vi "RunStep.vi"(4 "syringe_volume_uL":dbl=1000.0, 5 "MessageQueues":T1, 6 "Experiment":string[][](array[string]), 7 "Current Step 2":refnum<vi>, 8 "Pump Class":refnum<k24>, 9 "Bias":refnum<vi>, 10 "TimeTrace":refnum<vi>, 11 "Analyte":refnum<vi>) -> ()   [LabVIEW 2024]
uses:
  MessageQueues.ctl
  <vilib>/httpClient/ClientHandle.ctl
  E:/CodeProjects/DEMPbot/ChannelAutomatorR2/PumpAdapter.exe
  PumpAdapter.exe
  <vilib>/httpClient/LabVIEWHTTPClient.lvlib
panel:
  out "DispenseToCellLimited2":string
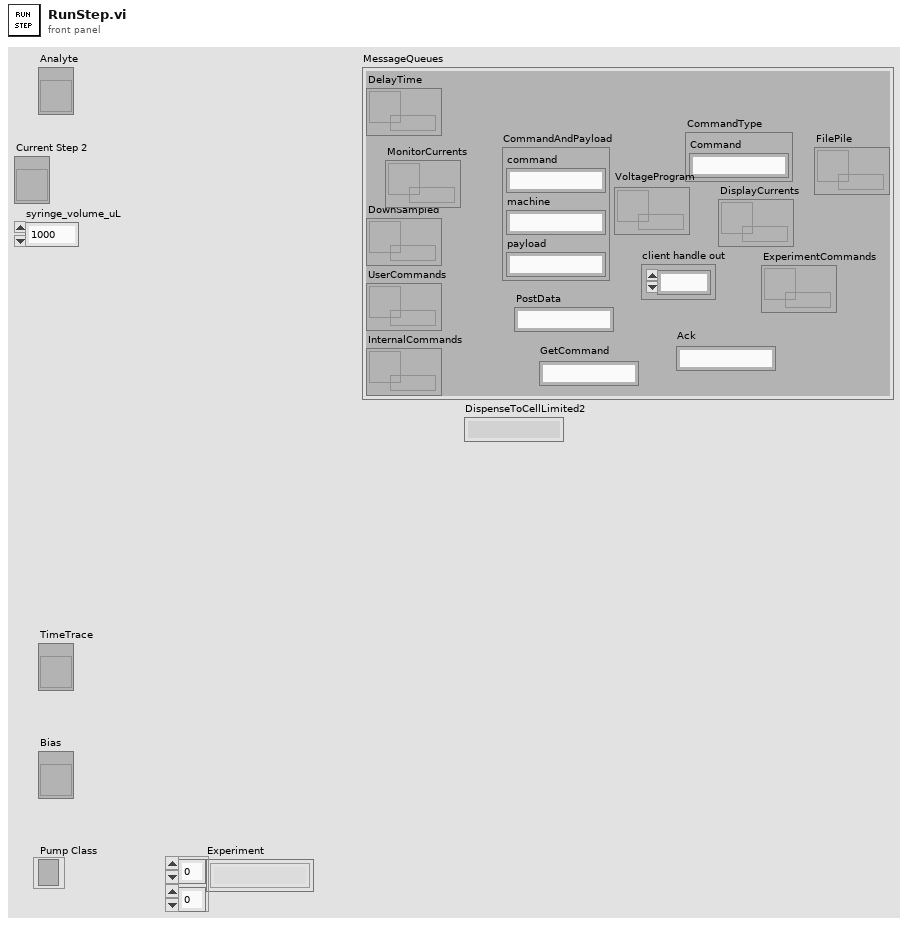
[diagram p1: front panel]
types:
  T1 = typedef "MessageQueues.ctl" = cluster{"DelayTime":refnum<queue>, "DownSampled":refnum<queue>, "UserCommands":refnum<queue>, "InternalCommands":refnum<queue>, "CommandType":cluster{"Command":string}, "CommandAndPayload":cluster{"command":string, "machine":string, "payload":string}, "client handle out":T2, "PostData":string, "GetCommand":string, "Ack":string, "VoltageProgram":refnum<queue>, "ExperimentCommands":refnum<queue>, "DisplayCurrents":refnum<queue>, "MonitorCurrents":refnum<queue>, "FilePile":refnum<queue>}
  T2 = typedef "LabVIEWHTTPClient.lvlib/ClientHandle.ctl" = refnum<k1>
  T3 = cluster{"Step":string, "Push":string, "Analyte1":string, "Volume1":dbl, "Analyte2":string, "Measurement":string, "Volume2":dbl, "Speed1":dbl, "Speed2":dbl, "MinTime":dbl, "Bias":dbl, "Slew":dbl, "Parameter1":string, "Parameter2":string}
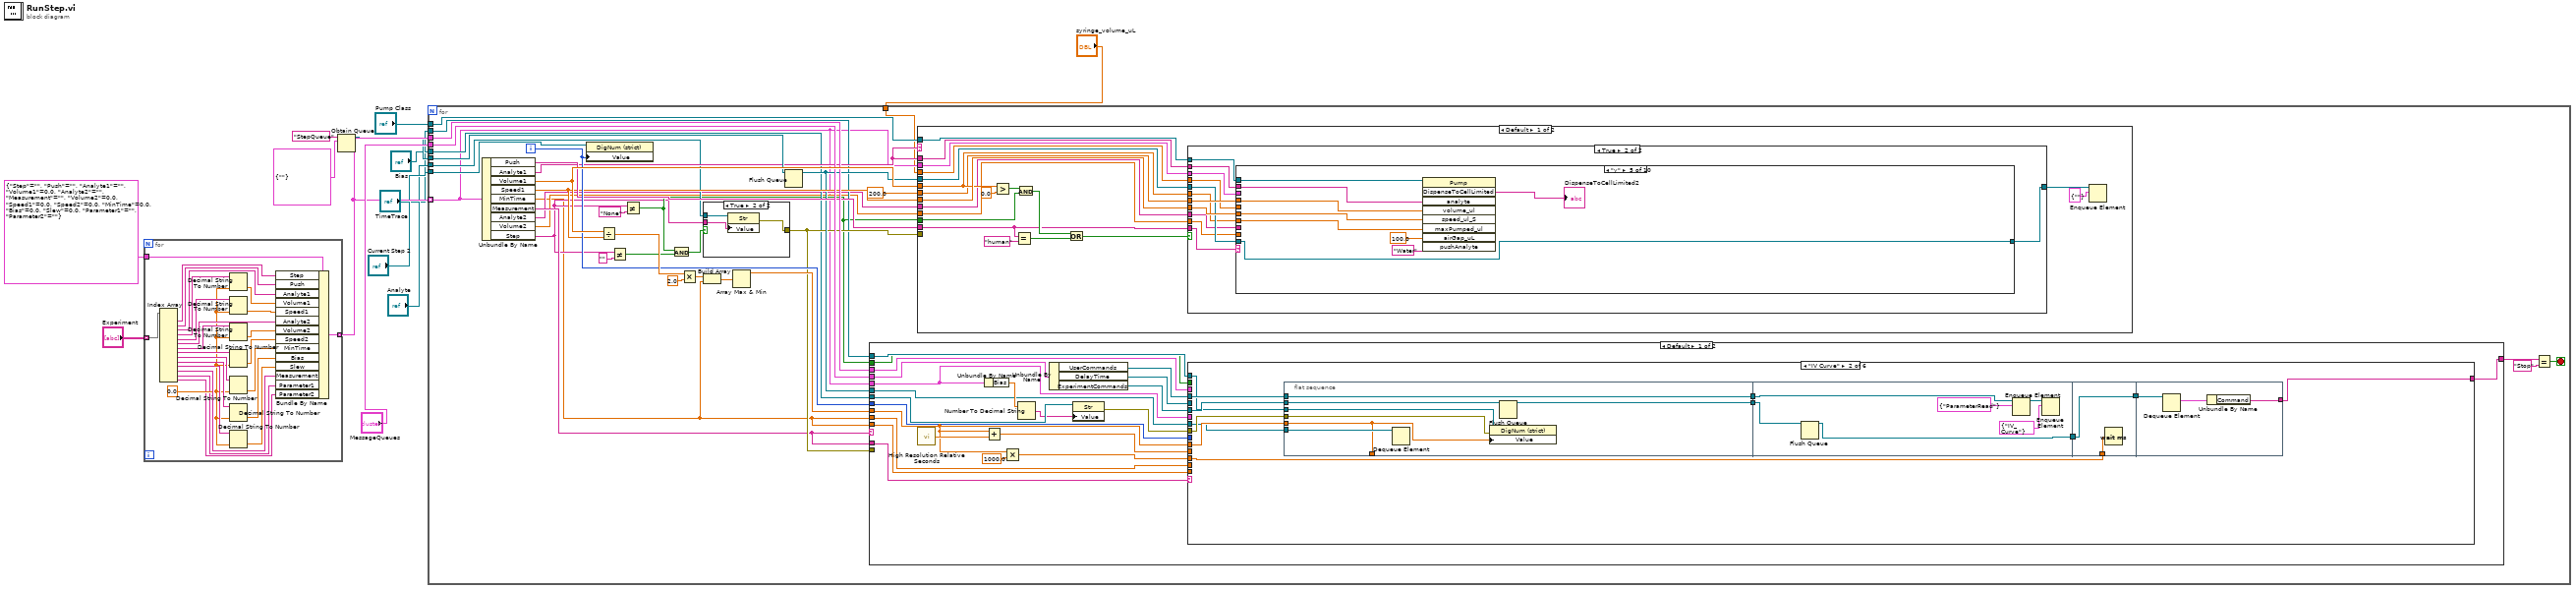
[diagram p0: block diagram]
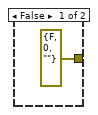
[diagram p2: hidden frame]
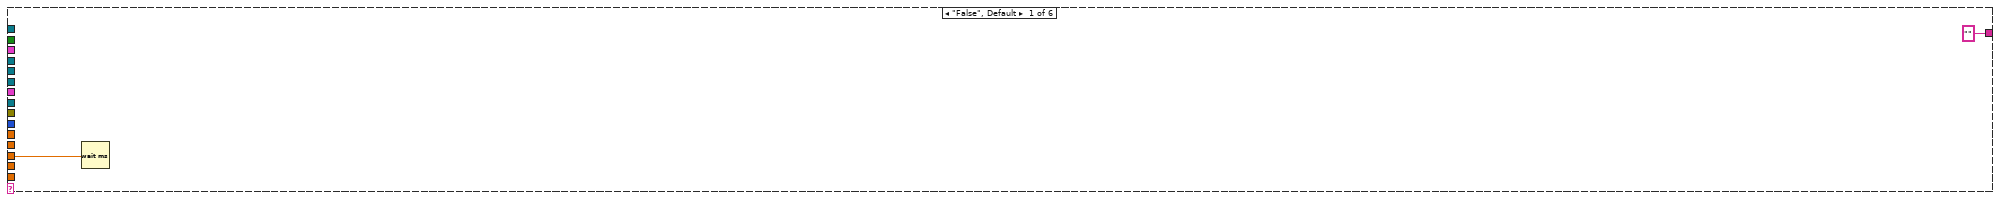
[diagram p3: hidden frame]
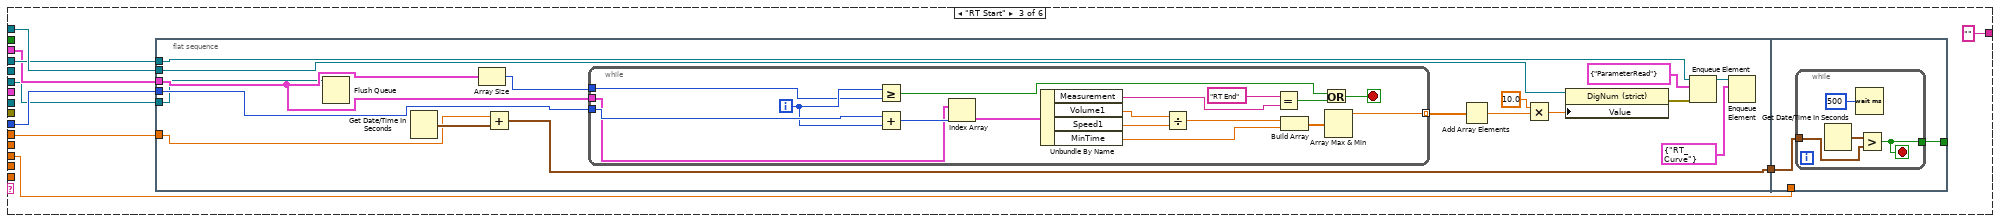
[diagram p4: hidden frame]
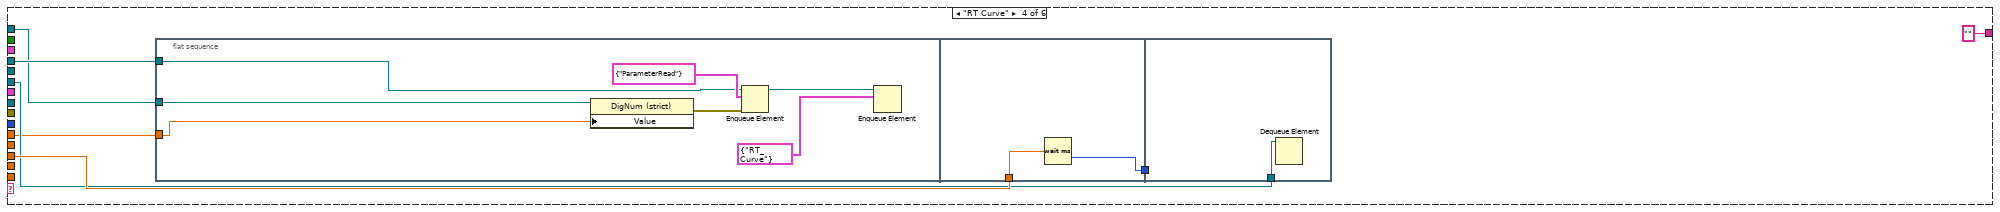
[diagram p5: hidden frame]
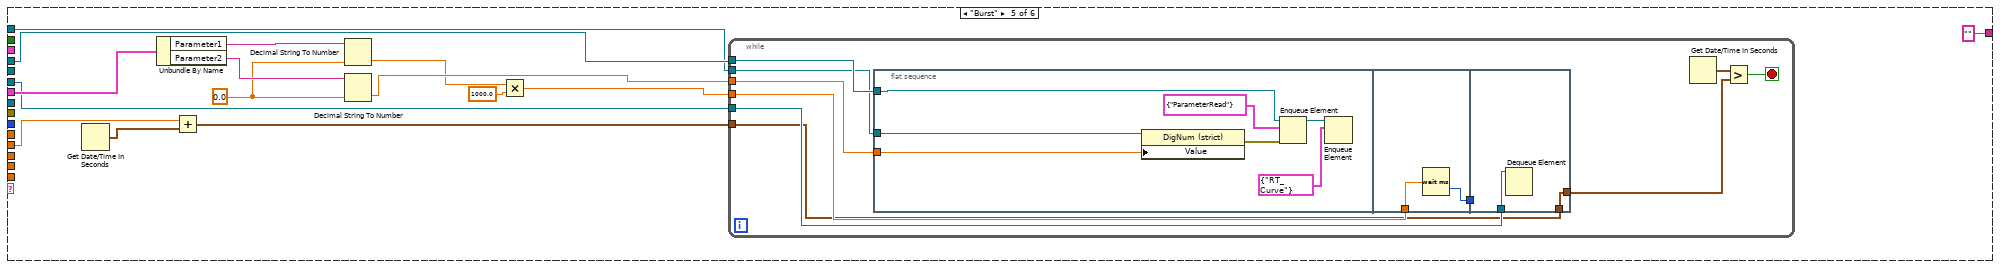
[diagram p6: hidden frame]
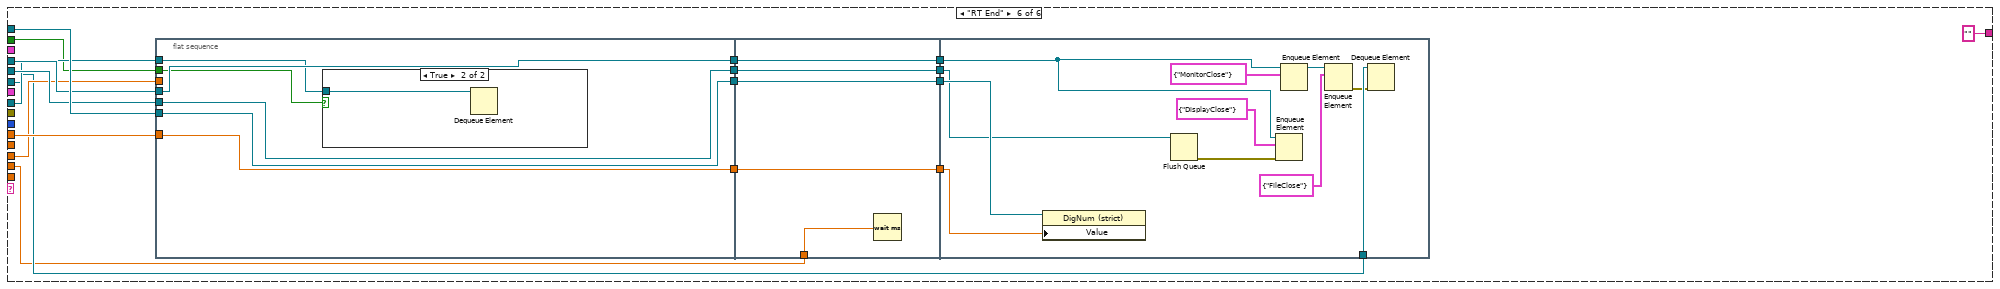
[diagram p7: hidden frame]
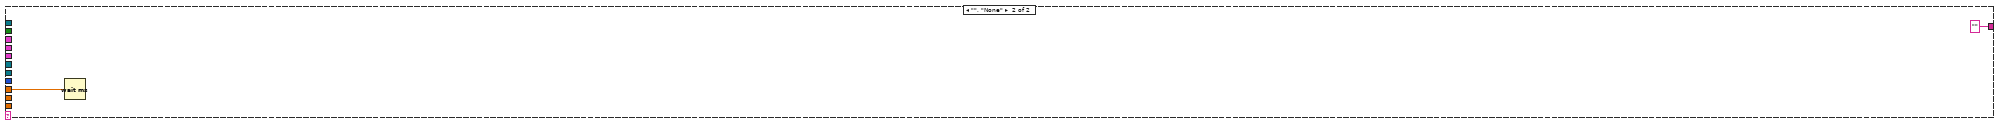
[diagram p9: hidden frame]
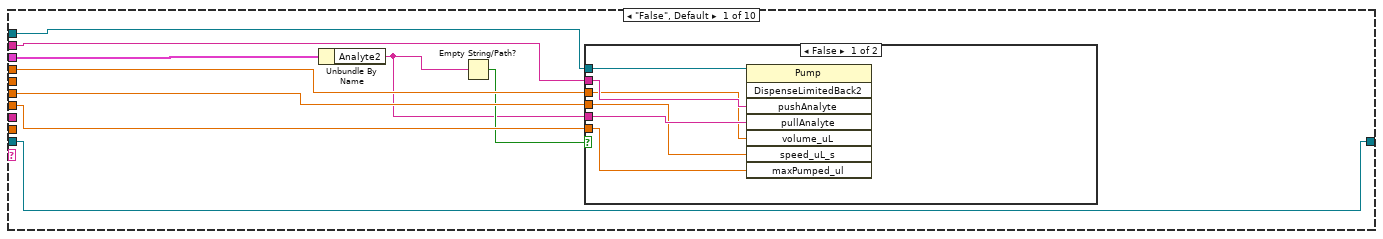
[diagram p11: hidden frame]
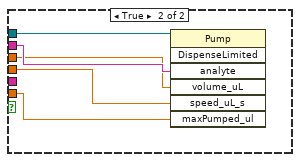
[diagram p12: hidden frame]
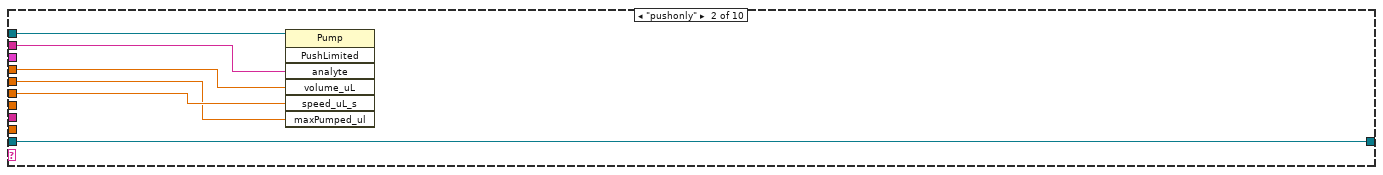
[diagram p13: hidden frame]
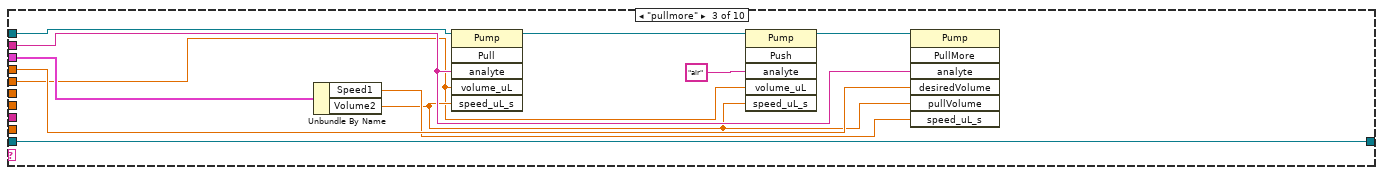
[diagram p14: hidden frame]
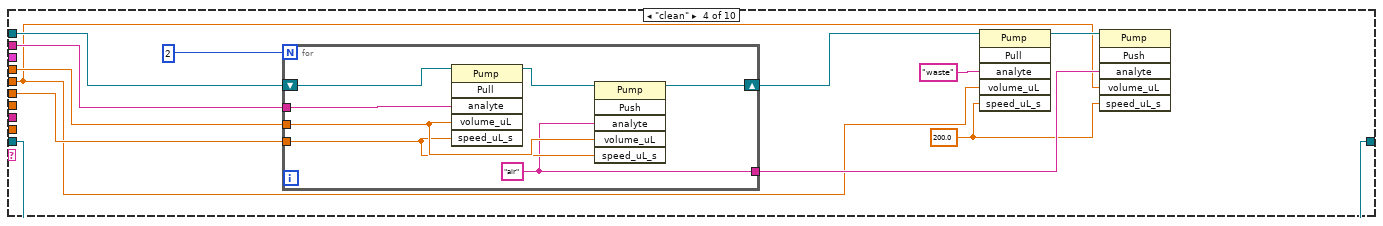
[diagram p15: hidden frame]
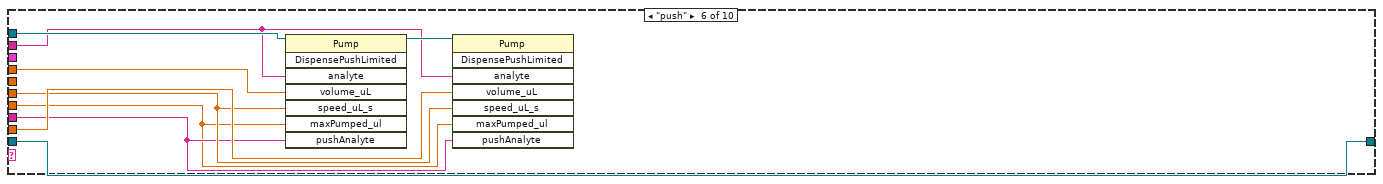
[diagram p16: hidden frame]
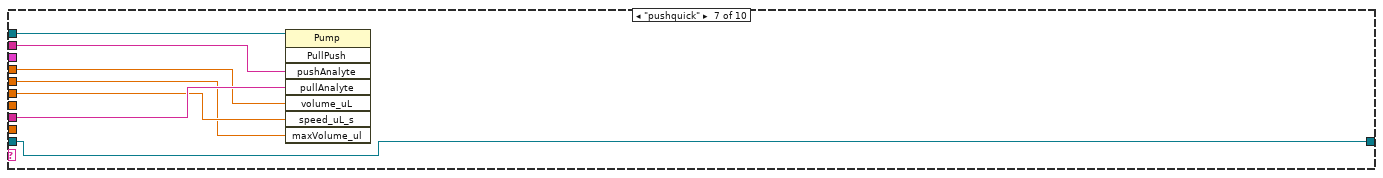
[diagram p17: hidden frame]
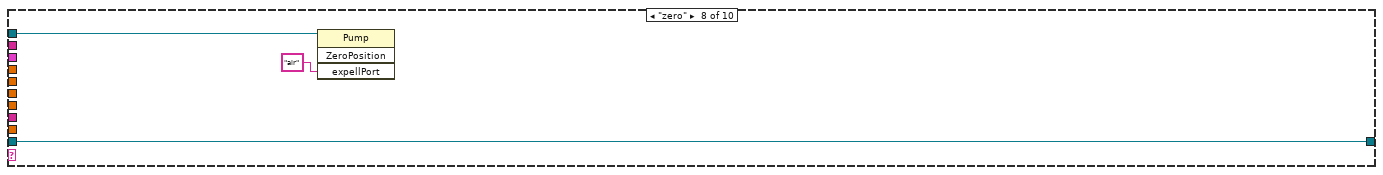
[diagram p18: hidden frame]
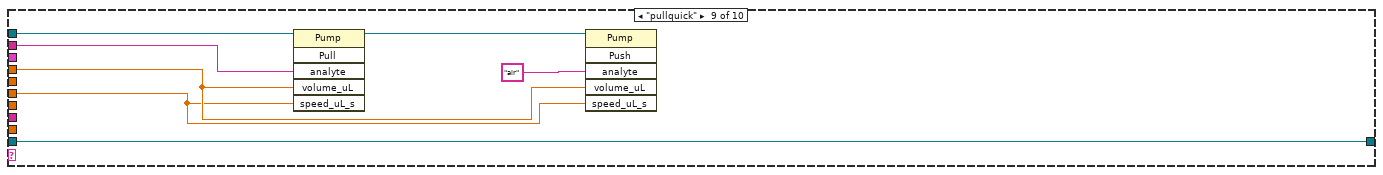
[diagram p19: hidden frame]
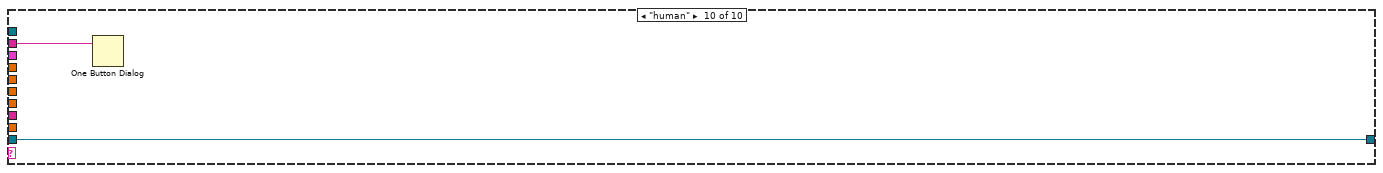
[diagram p20: hidden frame]
diagram:
  n1 = for {
    tunnel: T3 {"Step"="", "Push"="", "Analyte1"="", "Volume1"=0.0, "Analyte2"="", "Measurement"="", "Volume2"=0.0, "Speed1"=0.0, "Speed2"=0.0, "MinTime"=0.0, "Bias"=0.0, "Slew"=0.0, "Parameter1"="", "Parameter2"=""} -> [w19]
    tunnel: "Experiment" -> [w17] mode=indexing
    tunnel: [w16] -> w10 mode=indexing
    w20 = 0.0
    n2 = Index Array(array=w17) -> (element #1=w38:string, element #2=w37:string, element #3=w30:string, element #4=w36:string, element #5=w35:string, element #6=w34:string, element #7=w33:string, element #8=w32:string, element #9=w31:string, element #10=w28:string, element #11=w24:string, element #12=w23:string, element #13=w15:string, element #14=w14:string)  [unwired: 14 in]
    n3 = Decimal String To Number(string=w36, default (0L)=w20) -> (number=w25:dbl)  [unwired: 1 in, 1 out]
    n4 = Decimal String To Number(string=w35, default (0L)=w20) -> (number=w26:dbl)  [unwired: 1 in, 1 out]
    n5 = Decimal String To Number(string=w33, default (0L)=w20) -> (number=w27:dbl)  [unwired: 1 in, 1 out]
    n6 = Decimal String To Number(string=w32, default (0L)=w20) -> (number=w29:dbl)  [unwired: 1 in, 1 out]
    n7 = Decimal String To Number(string=w31, default (0L)=w20) -> (number=w18:dbl)  [unwired: 1 in, 1 out]
    n8 = Decimal String To Number(string=w28, default (0L)=w20) -> (number=w22:dbl)  [unwired: 1 in, 1 out]
    n9 = Decimal String To Number(string=w24, default (0L)=w20) -> (number=w21:dbl)  [unwired: 1 in, 1 out]
    n10 = Bundle By Name(cluster=w19, "Step"=w38, "Push"=w37, "Analyte1"=w30, "Volume1"=w25, "Speed1"=w26, "Analyte2"=w34, "Volume2"=w27, "Speed2"=w29, "MinTime"=w18, "Bias"=w22, "Slew"=w21, "Measurement"=w23, "Parameter1"=w15, "Parameter2"=w14) -> (w16:T3)
  }
  n11 = Obtain Queue(name (unnamed)="StepQueue", element data type=cluster{string} {""}) -> (queue out=w7:refnum<queue>)  [unwired: 3 in, 2 out]
  n12 = for {
    tunnel: "MessageQueues" -> [w70]
    tunnel: w10 -> [w66]
    tunnel: w10 -> [w43] mode=indexing
    tunnel: w7 -> [w62]
    tunnel: "Current Step 2" -> [w57]
    tunnel: "Analyte" -> [w56]
    tunnel: "Pump Class" -> [w55]
    tunnel: "Bias" -> [w54]
    tunnel: "TimeTrace" -> [w53]
    tunnel: "syringe_volume_uL" -> [w39]
    i -> [w65]
    stop <- w68 stop-if-true
    n13 = Unbundle By Name(w43) -> ("Push"=w64:string, "Analyte1"=w60:string, "Volume1"=w72:dbl, "Speed1"=w63:dbl, "MinTime"=w42:dbl, "Measurement"=w51:string, "Analyte2"=w50:string, "Volume2"=w49:dbl, "Step"=w44:string)
    n14 = property class="DigNum (strict)"(reference=w57, "Value"=w65) -> ()  [unwired: 1 in, 2 out]
    n15 = Divide(x=w72, y=w63) -> (x/y=w71:dbl)
    n16 = Not Equal?(x=w44, y="") -> (x != y?=w46:bool)
    n17 = Not Equal?(x=w44, y="None") -> (x != y?=w52:bool)
    n18 = And(x=w52, y=w46) -> (x .and. y?=w47:bool)
    n19 = Multiply(x=w71, y=2.0) -> (x*y=w41:dbl)
    n20 = case shown="True" w47 {
      tunnel: w56 -> [_ w78]
      tunnel: w44 -> [_ w77]
      tunnel: [errorcluster {"status"=FALSE, "code"=0, "source"=""} ("error out") w76] -> w58
      frame False {
      }
      frame True {
        n21 = property class="Str"(reference=w78, "Value"=w77) -> (error out=w76:errorcluster)  [unwired: 1 in, 1 out]
      }
    }
    n22 = Build Array(w41, w42) -> (w73:dbl[])
    n23 = Array Max & Min(array=w73) -> (max value=w74:dbl)  [unwired: 3 out]
    n24 = Flush Queue(queue=w62) -> (queue out=w61:refnum<queue>)  [unwired: 1 in, 2 out]
    n25 = case shown="Default" w51 {
      tunnel: w70 -> [w101 _]
      tunnel: w51 -> [w100 _]
      tunnel: w74 -> [w85 w278]
      tunnel: w43 -> [w98 _]
      tunnel: w53 -> [w94 _]
      tunnel: w54 -> [w96 _]
      tunnel: [w89 "" ("Command")] -> w67
      tunnel: w66 -> [w87 _]
      tunnel: w65 -> [w86 _]
      tunnel: w61 -> [w82 _]
      tunnel: w42 -> [w81 _]
      tunnel: w58 -> [_ _]
      tunnel: w52 -> [w80 _]
      tunnel: w42 -> [w79 _]
      frame Default {
        n26 = call <vilib>:"High Resolution Relative Seconds.vi"() -> ("relative seconds"=w91:dbl)
        n27 = Unbundle By Name(w98) -> ("Bias"=w97:dbl)
        n28 = Add(x=w85, y=w91) -> (x+y=w90:dbl)
        n29 = Multiply(x=w85, y=1000.0) -> (x*y=w83:dbl)
        n30 = Number To Decimal String(number=w97) -> (decimal integer string=w95:string)  [unwired: 1 in]
        n31 = Unbundle By Name(w101) -> ("UserCommands"=w99:refnum<queue>, "DelayTime"=w92:refnum<queue>, "ExperimentCommands"=w88:refnum<queue>)
        n32 = property class="Str"(reference=w96, "Value"=w95) -> (error out=w93:errorcluster)  [unwired: 1 in, 1 out]
        n33 = case shown="\"IV Curve\"" w100 {
          tunnel: w99 -> [_ w115 w141 w188 w209 w250]
          tunnel: w98 -> [_ _ _ _ w214 _]
          tunnel: w94 -> [_ w110 w142 w184 w203 w253]
          tunnel: w93 -> [_ w109 _ _ _ _]
          tunnel: w92 -> [_ _ _ _ _ w251]
          tunnel: w90 -> [_ _ _ _ w202 _]
          tunnel: ["" ("Command") w114 "" ("Command") "" ("Command") "" ("Command") "" ("Command")] -> w89
          tunnel: w88 -> [_ w113 w134 w185 w204 w238]
          tunnel: w85 -> [_ w108 w135 w183 _ w249]
          tunnel: w87 -> [_ _ w139 _ _ _]
          tunnel: w86 -> [_ _ w138 _ _ _]
          tunnel: w83 -> [w102 w104 w137 w187 _ w248]
          tunnel: w82 -> [_ w107 _ _ _ w247]
          tunnel: w81 -> [_ _ _ _ _ _]
          tunnel: w80 -> [_ _ _ _ _ w237]
          tunnel: w79 -> [_ _ _ _ _ w236]
          frame "False", Default {
            n34 = Wait (ms)(milliseconds to wait=w102) -> ()  [unwired: 1 out]
          }
          frame "IV Curve" {
            n35 = flat-sequence {
              tunnel: w113 -> [w121]
              tunnel: w115 -> [w122]
              tunnel: [w122] -> w112
              tunnel: [w117] -> w111
              tunnel: w110 -> [w120]
              tunnel: w109 -> [w119]
              tunnel: w108 -> [w116]
              tunnel: w107 -> [w118]
              tunnel: [w116] -> _
              tunnel: w112 -> [w128]
              tunnel: w111 -> [w124]
              tunnel: [w123] -> w106
              tunnel: w106 -> [w130]
              tunnel: [w130] -> w105
              tunnel: w104 -> [w129]
              tunnel: [w131] -> w114
              tunnel: w105 -> [w132]
              frame #0 {
                n36 = Dequeue Element(queue=w118) -> ()  [unwired: 2 in, 4 out]
                n37 = property class="DigNum (strict)"(reference=w120, error in=w119, "Value"=w116) -> ()  [unwired: 2 out]
                n38 = Flush Queue(queue=w121) -> (queue out=w117:refnum<queue>)  [unwired: 1 in, 2 out]
              }
              frame #1 {
                n39 = Flush Queue(queue=w124) -> (queue out=w123:refnum<queue>)  [unwired: 1 in, 2 out]
                n40 = Enqueue Element(queue=w128, element=cluster{"Command":string} {"Command"="ParameterRead"}) -> (queue out=w127:refnum<queue>)  [unwired: 2 in, 2 out]
                n41 = Enqueue Element(queue=w127, element=cluster{"Command":string} {"Command"="IV_Curve"}) -> ()  [unwired: 2 in, 3 out]
              }
              frame #2 {
                n42 = Wait (ms)(milliseconds to wait=w129) -> ()  [unwired: 1 out]
              }
              frame #3 {
                n43 = Dequeue Element(queue=w132) -> (element=w133:cluster{"Command":string})  [unwired: 2 in, 3 out]
                n44 = Unbundle By Name(w133) -> ("Command"=w131:string)
              }
            }
          }
          frame "RT Start" {
            n45 = flat-sequence {
              tunnel: w142 -> [w156]
              tunnel: w141 -> [w155]
              tunnel: w139 -> [w153]
              tunnel: w138 -> [w154]
              tunnel: [w145] -> w136
              tunnel: w135 -> [w144]
              tunnel: w134 -> [w143]
              tunnel: w137 -> [_]
              tunnel: w136 -> [w178]
              tunnel: [w177] -> _
              frame #0 {
                n46 = Flush Queue(queue=w143) -> ()  [unwired: 1 in, 3 out]
                n47 = Get Date/Time In Seconds() -> (seconds since 1Jan1904=w146:timestamp)
                n48 = Array Size(array=w153) -> (size(s)=w152:i32)
                n49 = Add(x=w144, y=w146) -> (x+y=w145:timestamp)
                n50 = while {
                  tunnel: w154 -> [w176]
                  tunnel: w153 -> [w174]
                  tunnel: w152 -> [w171]
                  tunnel: [w160] -> w151 mode=indexing
                  i -> [w172]
                  stop <- w169 stop-if-true
                  n51 = Greater Or Equal?(x=w172, y=w171) -> (x >= y?=w170:bool)
                  n52 = Add(x=w176, y=w172) -> (x+y=w175:i32)
                  n53 = Index Array(array=w174, index=w175) -> (element=w173:T3)
                  n54 = Unbundle By Name(w173) -> ("Measurement"=w168:string, "Volume1"=w165:dbl, "Speed1"=w164:dbl, "MinTime"=w162:dbl)
                  n55 = Divide(x=w165, y=w164) -> (x/y=w163:dbl)
                  n56 = Equal?(x="RT End", y=w168) -> (x = y?=w166:bool)
                  n57 = Build Array(w163, w162) -> (w161:dbl[])
                  n58 = Or(x=w170, y=w166) -> (x .or. y?=w169:bool)
                  n59 = Array Max & Min(array=w161) -> (max value=w160:dbl)  [unwired: 3 out]
                }
                n60 = Add Array Elements(numeric array=w151) -> (sum=w150:dbl)
                n61 = Multiply(x=10.0, y=w150) -> (x*y=w148:dbl)
                n62 = property class="DigNum (strict)"(reference=w156, "Value"=w148) -> (error out=w149:errorcluster)  [unwired: 1 in, 1 out]
                n63 = Enqueue Element(queue=w155, element=cluster{"Command":string} {"Command"="ParameterRead"}, error in (no error)=w149) -> (queue out=w159:refnum<queue>)  [unwired: 1 in, 2 out]
                n64 = Enqueue Element(queue=w159, element=cluster{"Command":string} {"Command"="RT_Curve"}) -> ()  [unwired: 2 in, 3 out]
              }
              frame #1 {
                n65 = while {
                  tunnel: w178 -> [w180]
                  tunnel: [w179] -> w177
                  stop <- w179 stop-if-true
                  n66 = Get Date/Time In Seconds() -> (seconds since 1Jan1904=w181:timestamp)
                  n67 = Wait (ms)(milliseconds to wait=u32 500) -> ()  [unwired: 1 out]
                  n68 = Greater?(x=w181, y=w180) -> (0:w179:bool)
                }
              }
            }
          }
          frame "RT Curve" {
            n69 = flat-sequence {
              tunnel: w188 -> [w193]
              tunnel: w183 -> [w191]
              tunnel: w184 -> [w190]
              tunnel: w187 -> [w197]
              tunnel: [w198] -> w186
              tunnel: w186 -> [_]
              tunnel: w185 -> [w199]
              frame #0 {
                n70 = property class="DigNum (strict)"(reference=w190, "Value"=w191) -> (error out=w192:errorcluster)  [unwired: 1 in, 1 out]
                n71 = Enqueue Element(queue=w193, element=cluster{"Command":string} {"Command"="ParameterRead"}, error in (no error)=w192) -> (queue out=w196:refnum<queue>)  [unwired: 1 in, 2 out]
                n72 = Enqueue Element(queue=w196, element=cluster{"Command":string} {"Command"="RT_Curve"}) -> ()  [unwired: 2 in, 3 out]
              }
              frame #1 {
                n73 = Wait (ms)(milliseconds to wait=w197) -> (millisecond timer value=w198:u32)
              }
              frame #2 {
                n74 = Dequeue Element(queue=w199) -> ()  [unwired: 2 in, 4 out]
              }
            }
          }
          frame "Burst" {
            w211 = 0.0
            n75 = Get Date/Time In Seconds() -> (seconds since 1Jan1904=w201:timestamp)
            n76 = Unbundle By Name(w214) -> ("Parameter1"=w213:string, "Parameter2"=w212:string)
            n77 = Add(x=w202, y=w201) -> (x+y=w200:timestamp)
            n78 = Decimal String To Number(string=w213, default (0L)=w211) -> (number=w207:dbl)  [unwired: 1 in, 1 out]
            n79 = Decimal String To Number(string=w212, default (0L)=w211) -> (number=w208:dbl)  [unwired: 1 in, 1 out]
            n80 = Multiply(x=w207, y=1000.0) -> (x*y=w205:dbl)
            n81 = while {
              tunnel: w209 -> [w223]
              tunnel: w208 -> [w222]
              tunnel: w205 -> [w221]
              tunnel: w204 -> [w220]
              tunnel: w203 -> [w219]
              tunnel: w200 -> [w216]
              stop <- w217 stop-if-true
              n82 = flat-sequence {
                tunnel: w219 -> [w227]
                tunnel: w223 -> [w226]
                tunnel: w222 -> [w225]
                tunnel: w221 -> [w232]
                tunnel: [w233] -> w224
                tunnel: w224 -> [_]
                tunnel: w220 -> [w235]
                tunnel: [w234] -> w215
                tunnel: w216 -> [w234]
                frame #0 {
                  n83 = property class="DigNum (strict)"(reference=w227, "Value"=w225) -> (error out=w228:errorcluster)  [unwired: 1 in, 1 out]
                  n84 = Enqueue Element(queue=w226, element=cluster{"Command":string} {"Command"="ParameterRead"}, error in (no error)=w228) -> (queue out=w231:refnum<queue>)  [unwired: 1 in, 2 out]
                  n85 = Enqueue Element(queue=w231, element=cluster{"Command":string} {"Command"="RT_Curve"}) -> ()  [unwired: 2 in, 3 out]
                }
                frame #1 {
                  n86 = Wait (ms)(milliseconds to wait=w232) -> (millisecond timer value=w233:u32)
                }
                frame #2 {
                  n87 = Dequeue Element(queue=w235) -> ()  [unwired: 2 in, 4 out]
                }
              }
              n88 = Get Date/Time In Seconds() -> (seconds since 1Jan1904=w218:timestamp)
              n89 = Greater?(x=w218, y=w215) -> (0:w217:bool)
            }
          }
          frame "RT End" {
            n90 = flat-sequence {
              tunnel: w248 -> [_]
              tunnel: w249 -> [w256]
              tunnel: w250 -> [w257]
              tunnel: w251 -> [w258]
              tunnel: w253 -> [w259]
              tunnel: [w259] -> w246
              tunnel: [w258] -> w244
              tunnel: [w257] -> w242
              tunnel: [w256] -> w240
              tunnel: w247 -> [w255]
              tunnel: w237 -> [w254]
              tunnel: w246 -> [w265]
              tunnel: [w265] -> w245
              tunnel: w244 -> [w264]
              tunnel: [w264] -> w243
              tunnel: w242 -> [w263]
              tunnel: [w263] -> w241
              tunnel: w240 -> [w262]
              tunnel: [w262] -> w239
              tunnel: w236 -> [w261]
              tunnel: w245 -> [w275]
              tunnel: w243 -> [w274]
              tunnel: w241 -> [w271]
              tunnel: w239 -> [w269]
              tunnel: w238 -> [w267]
              frame #0 {
                n91 = case shown="True" w254 {
                  tunnel: w255 -> [_ w260]
                  frame False {
                  }
                  frame True {
                    n92 = Dequeue Element(queue=w260) -> ()  [unwired: 2 in, 4 out]
                  }
                }
              }
              frame #1 {
                n93 = Wait (ms)(milliseconds to wait=w261) -> ()  [unwired: 1 out]
              }
              frame #2 {
                n94 = property class="DigNum (strict)"(reference=w275, "Value"=w269) -> ()  [unwired: 1 in, 2 out]
                n95 = Flush Queue(queue=w274) -> (error out=w268:errorcluster)  [unwired: 1 in, 2 out]
                n96 = Enqueue Element(queue=w271, element=cluster{"Command":string} {"Command"="DisplayClose"}, error in (no error)=w268) -> ()  [unwired: 1 in, 3 out]
                n97 = Enqueue Element(queue=w271, element=cluster{"Command":string} {"Command"="MonitorClose"}) -> (queue out=w276:refnum<queue>)  [unwired: 2 in, 2 out]
                n98 = Enqueue Element(queue=w276, element=cluster{"Command":string} {"Command"="FileClose"}) -> (error out=w266:errorcluster)  [unwired: 2 in, 2 out]
                n99 = Dequeue Element(queue=w267, error in (no error)=w266) -> ()  [unwired: 1 in, 4 out]
              }
            }
          }
        }
      }
      frame "", "None" {
        n100 = Wait (ms)(milliseconds to wait=w278) -> ()  [unwired: 1 out]
      }
    }
    n101 = case shown="Default" w60 {
      tunnel: w55 -> [w297 _]
      tunnel: w60 -> [w284 _]
      tunnel: w72 -> [w295 _]
      tunnel: w64 -> [w281 _]
      tunnel: w63 -> [w298 _]
      tunnel: w61 -> [w294 _]
      tunnel: w52 -> [w289 _]
      tunnel: w58 -> [_ _]
      tunnel: w50 -> [w288 _]
      tunnel: w49 -> [w287 _]
      tunnel: 200.0 ("maxPumped_ul") -> [w286 _]
      tunnel: w43 -> [w280 _]
      tunnel: w39 -> [w279 _]
      frame Default {
        n102 = Greater?(x=w295, y=0.0) -> (0:w291:bool)
        n103 = Equal?(x=w281, y="human") -> (x = y?=w283:bool)
        n104 = And(x=w291, y=w289) -> (x .and. y?=w290:bool)
        n105 = Or(x=w290, y=w283) -> (x .or. y?=w285:bool)
        n106 = case shown="True" w285 {
          tunnel: w281 -> [_ w311]
          tunnel: w284 -> [_ w310]
          tunnel: w298 -> [_ w309]
          tunnel: w297 -> [_ w308]
          tunnel: w295 -> [_ w307]
          tunnel: w294 -> [w299 w306]
          tunnel: [w299 w305] -> w293
          tunnel: w288 -> [_ w304]
          tunnel: w287 -> [_ w303]
          tunnel: w286 -> [_ w302]
          tunnel: w280 -> [_ w301]
          tunnel: w279 -> [_ w300]
          frame False {
          }
          frame True {
            n107 = case shown="\"y\"" w311 {
              tunnel: w310 -> [w319 w336 w342 w359 w376 w378 w391 _ w401 w403]
              tunnel: w309 -> [w317 w334 _ w357 w375 w380 w388 _ w396 _]
              tunnel: w308 -> [w320 w337 w348 w360 w374 w385 w392 w395 w402 _]
              tunnel: w307 -> [w318 w335 w347 w358 w373 w383 w389 _ w397 _]
              tunnel: [w316 w333 w344 w351 w372 w384 w387 w393 w400 w404] -> w305
              tunnel: w306 -> [w316 w333 w344 w351 w372 w384 w387 w393 w400 w404]
              tunnel: w304 -> [_ _ _ _ _ w379 w390 _ _ _]
              tunnel: w303 -> [_ _ _ _ _ w381 _ _ _ _]
              tunnel: w302 -> [w315 _ _ _ w368 w377 _ _ _ _]
              tunnel: w301 -> [w314 _ w346 _ _ _ _ _ _ _]
              tunnel: w300 -> [_ w332 w338 w349 _ _ w386 _ _ _]
              frame "False", Default {
                n108 = Unbundle By Name(w314) -> ("Analyte2"=w312:string)
                n109 = Empty String/Path?(string/path=w312) -> (empty?=w313:bool)
                n110 = case shown="False" w313 {
                  tunnel: w320 -> [w326 w331]
                  tunnel: w319 -> [w325 w330]
                  tunnel: w318 -> [w323 w329]
                  tunnel: w317 -> [w322 w328]
                  tunnel: w315 -> [w321 w327]
                  tunnel: w312 -> [w324 _]
                  frame False {
                    n111 = invoke class="Pump" method="DispenseLimitedBack2"(reference=w326, "pushAnalyte"=w325, "pullAnalyte"=w324, "volume_uL"=w323, "speed_uL_s"=w322, "maxPumped_ul"=w321) -> ()  [unwired: 2 in, 8 out]
                  }
                  frame True {
                    n112 = invoke class="Pump" method="DispenseLimited"(reference=w331, "analyte"=w330, "volume_uL"=w329, "speed_uL_s"=w328, "maxPumped_ul"=w327) -> ()  [unwired: 2 in, 7 out]
                  }
                }
              }
              frame "pushonly" {
                n113 = invoke class="Pump" method="PushLimited"(reference=w337, "analyte"=w336, "volume_uL"=w335, "speed_uL_s"=w334, "maxPumped_ul"=w332) -> ()  [unwired: 2 in, 7 out]
              }
              frame "pullmore" {
                n114 = Unbundle By Name(w346) -> ("Speed1"=w345:dbl, "Volume2"=w339:dbl)
                n115 = invoke class="Pump" method="Pull"(reference=w348, "analyte"=w342, "volume_uL"=w338, "speed_uL_s"=w339) -> (reference out=w343:refnum<k24>)  [unwired: 2 in, 5 out]
                n116 = invoke class="Pump" method="Push"(reference=w343, "analyte"="air", "volume_uL"=w338, "speed_uL_s"=w339) -> (reference out=w341:refnum<k24>)  [unwired: 2 in, 5 out]
                n117 = invoke class="Pump" method="PullMore"(reference=w341, "analyte"=w342, "desiredVolume"=w347, "pullVolume"=w339, "speed_uL_s"=w345) -> ()  [unwired: 2 in, 7 out]
              }
              frame "clean" {
                w352 = 200.0 ("speed_uL_s")
                n118 = for {
                  N: 2 -> [_]
                  tunnel: w359 -> [w366]
                  tunnel: w358 -> [w364]
                  tunnel: w357 -> [w363]
                  tunnel: [w361] -> w353
                  shift-right: [w362] -> w356
                  shift-left: w360 -> [w367]
                  w361 = "air" ("analyte")
                  n119 = invoke class="Pump" method="Pull"(reference=w367, "analyte"=w366, "volume_uL"=w364, "speed_uL_s"=w363) -> (reference out=w365:refnum<k24>)  [unwired: 2 in, 5 out]
                  n120 = invoke class="Pump" method="Push"(reference=w365, "analyte"=w361, "volume_uL"=w364, "speed_uL_s"=w363) -> (reference out=w362:refnum<k24>)  [unwired: 2 in, 5 out]
                }
                n121 = invoke class="Pump" method="Pull"(reference=w356, "analyte"="waste", "volume_uL"=w349, "speed_uL_s"=w352) -> (reference out=w354:refnum<k24>)  [unwired: 2 in, 5 out]
                n122 = invoke class="Pump" method="Push"(reference=w354, "analyte"=w353, "volume_uL"=w349, "speed_uL_s"=w352) -> ()  [unwired: 2 in, 6 out]
              }
              frame "y" {
                n123 = invoke class="Pump" method="DispenseToCellLimited"(reference=w374, "analyte"=w376, "volume_ul"=w373, "speed_ul_S"=w375, "maxPumped_ul"=w368, "airGap_uL"=100.0, "pushAnalyte"="Water") -> ("DispenseToCellLimited"=→"DispenseToCellLimited2":string)  [unwired: 2 in, 8 out]
              }
              frame "push" {
                n124 = invoke class="Pump" method="DispensePushLimited"(reference=w385, "analyte"=w378, "volume_uL"=w383, "speed_uL_s"=w380, "maxPumped_ul"=w377, "pushAnalyte"=w379) -> (reference out=w382:refnum<k24>)  [unwired: 2 in, 7 out]
                n125 = invoke class="Pump" method="DispensePushLimited"(reference=w382, "analyte"=w378, "volume_uL"=w381, "speed_uL_s"=w380, "maxPumped_ul"=w377, "pushAnalyte"=w379) -> ()  [unwired: 2 in, 8 out]
              }
              frame "pushquick" {
                n126 = invoke class="Pump" method="PullPush"(reference=w392, "pushAnalyte"=w391, "pullAnalyte"=w390, "volume_uL"=w389, "speed_uL_s"=w388, "maxVolume_ul"=w386) -> ()  [unwired: 2 in, 8 out]
              }
              frame "zero" {
                n127 = invoke class="Pump" method="ZeroPosition"(reference=w395, "expellPort"="air") -> ()  [unwired: 2 in, 4 out]
              }
              frame "pullquick" {
                n128 = invoke class="Pump" method="Pull"(reference=w402, "analyte"=w401, "volume_uL"=w397, "speed_uL_s"=w396) -> (reference out=w399:refnum<k24>)  [unwired: 2 in, 5 out]
                n129 = invoke class="Pump" method="Push"(reference=w399, "analyte"="air", "volume_uL"=w397, "speed_uL_s"=w396) -> ()  [unwired: 2 in, 6 out]
              }
              frame "human" {
                n130 = One Button Dialog(message=w403) -> ()  [unwired: 1 in, 1 out]
              }
            }
          }
        }
        n131 = Enqueue Element(queue=w293, element=cluster{string} {""}) -> ()  [unwired: 2 in, 3 out]
      }
      frame "", "None" {
      }
    }
    n132 = Equal?(x=w67, y="Stop") -> (x = y?=w68:bool)
  }
